vi "writeU64.vi"(8 "error in (no error)":errorcluster, 10 "Input":u64, 11 "ModbusBuffer in":refnum<class "ModbusBuffer.lvclass">) -> (0 "error out":errorcluster, 3 "ModbusBuffer out":refnum<class "ModbusBuffer.lvclass">)   [LabVIEW 2016, in "RTModbus.lvlib" / "ModbusBuffer.lvclass"]
uses:
  ModbusBuffer.lvclass
  ModbusBuffer.lvclass/ModbusBuffer.ctl
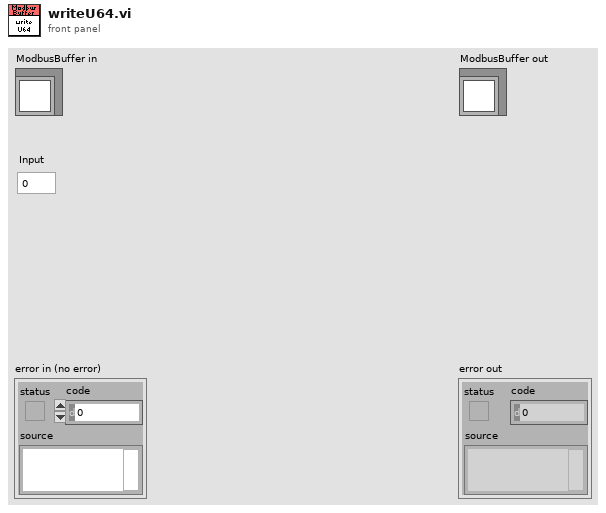
[diagram p1: front panel]
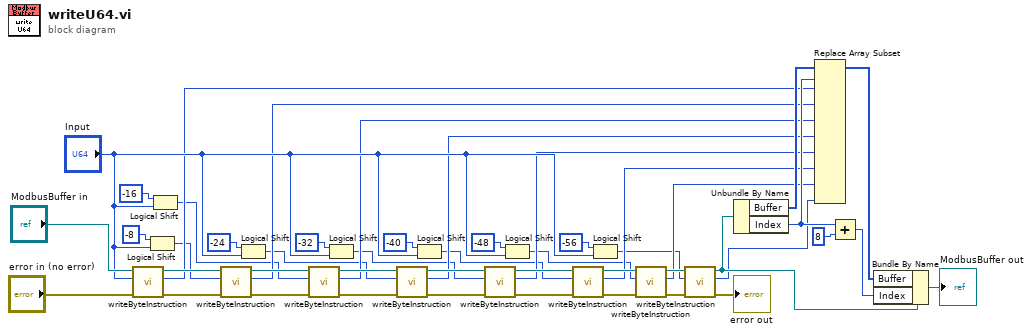
[diagram p0: block diagram]
diagram:
  n1 = call "writeByteInstruction.vi"("error in (no error)"="error in (no error)", "Input"="Input", "ModbusBuffer in"="ModbusBuffer in") -> ("error out"=w8:errorcluster, "Output"=w24:u16, "ModbusBuffer out"=w33:refnum<class "ModbusBuffer.lvclass">)  [unwired: 6 in]
  n2 = Logical Shift(y=i16 -8, x="Input") -> (x << y=w22:u64)
  n3 = Logical Shift(y=i16 -16, x="Input") -> (x << y=w21:u64)
  n4 = call "writeByteInstruction.vi"("error in (no error)"=w8, "Input"=w22, "ModbusBuffer in"=w33) -> ("error out"=w7:errorcluster, "Output"=w23:u16, "ModbusBuffer out"=w32:refnum<class "ModbusBuffer.lvclass">)  [unwired: 6 in]
  n5 = Logical Shift(y=i16 -24, x="Input") -> (x << y=w18:u64)
  n6 = call "writeByteInstruction.vi"("error in (no error)"=w7, "Input"=w21, "ModbusBuffer in"=w32) -> ("error out"=w6:errorcluster, "Output"=w20:u16, "ModbusBuffer out"=w31:refnum<class "ModbusBuffer.lvclass">)  [unwired: 6 in]
  n7 = Logical Shift(y=i16 -32, x="Input") -> (x << y=w17:u64)
  n8 = call "writeByteInstruction.vi"("error in (no error)"=w6, "Input"=w18, "ModbusBuffer in"=w31) -> ("error out"=w5:errorcluster, "Output"=w19:u16, "ModbusBuffer out"=w30:refnum<class "ModbusBuffer.lvclass">)  [unwired: 6 in]
  n9 = Logical Shift(y=i16 -40, x="Input") -> (x << y=w14:u64)
  n10 = call "writeByteInstruction.vi"("error in (no error)"=w5, "Input"=w17, "ModbusBuffer in"=w30) -> ("error out"=w4:errorcluster, "Output"=w16:u16, "ModbusBuffer out"=w29:refnum<class "ModbusBuffer.lvclass">)  [unwired: 6 in]
  n11 = Logical Shift(y=i16 -48, x="Input") -> (x << y=w13:u64)
  n12 = call "writeByteInstruction.vi"("error in (no error)"=w4, "Input"=w14, "ModbusBuffer in"=w29) -> ("error out"=w3:errorcluster, "Output"=w15:u16, "ModbusBuffer out"=w28:refnum<class "ModbusBuffer.lvclass">)  [unwired: 6 in]
  n13 = Logical Shift(y=i16 -56, x="Input") -> (x << y=w10:u64)
  n14 = call "writeByteInstruction.vi"("error in (no error)"=w3, "Input"=w13, "ModbusBuffer in"=w28) -> ("error out"=w2:errorcluster, "Output"=w12:u16, "ModbusBuffer out"=w27:refnum<class "ModbusBuffer.lvclass">)  [unwired: 6 in]
  n15 = call "writeByteInstruction.vi"("error in (no error)"=w2, "Input"=w10, "ModbusBuffer in"=w27) -> ("error out"=→"error out":errorcluster, "Output"=w11:u16, "ModbusBuffer out"=w26:refnum<class "ModbusBuffer.lvclass">)  [unwired: 6 in]
  n16 = Unbundle By Name(w26) -> ("Buffer"=w38:u16[], "Index"=w36:i32)
  n17 = Replace Array Subset(array=w38, new element #1=w24, index #1=w36, new element #2=w23, new element #3=w20, new element #4=w19, new element #5=w16, new element #6=w15, new element #7=w12, new element #8=w11) -> (w37:u16[])  [unwired: 7 in]
  n18 = Add(x=w36, y=8) -> (x+y=w46:i32)
  n19 = Bundle By Name(cluster=w26, "Buffer"=w37, "Index"=w46) -> (→"ModbusBuffer out":refnum<class "ModbusBuffer.lvclass">)
